vi "Process.vi"(8 "error in (no error)":errorcluster, 10 "Pound in":refnum<class "Pound.lvclass">, 11 "Qbus in":refnum<class "Qbus.lvclass">) -> (0 "error out":errorcluster)   [LabVIEW 2015]
doc: "The Analysis process calculates features and spectral bands, or trends, from waveforms the channels in a data group acquire. After these values are calculated, subsequent processes that evaluate their data to trigger alarms, file collections, and so on can operate."
uses:
  <vilib>/addons/Qbus/Qbus.lvclass
  <vilib>/NI/Software Watchdog/Pound/Pound.lvclass
  <vilib>/addons/InsightCM/Devices/Shared/VibrationAnalysisLoop/controls/Config.ctl
  <vilib>/addons/InsightCM/Devices/Shared/VibrationAnalysisLoop/controls/Group.ctl
  <vilib>/addons/InsightCM/Utilities/Analysis/Shared/controls/Channel.ctl
  <vilib>/addons/InsightCM/Utilities/Analysis/Shared/controls/Feature.ctl
  <vilib>/addons/InsightCM/Utilities/Analysis/Shared/controls/AmplitudeScale.ctl
  <vilib>/addons/InsightCM/Utilities/ChannelStatus/controls/RangeParams.ctl
  <vilib>/addons/InsightCM/Devices/Shared/VibrationAnalysisLoop/VibrationAnalysis.lvlib
  <vilib>/NI/Software Watchdog/Watchdog/Watchdog.lvclass
  <vilib>/addons/InsightCM/Devices/Shared/QbusHelpers/QbusHelper.lvlib
  <vilib>/addons/InsightCM/Devices/Shared/DataFlow/DataFlow.lvlib
  <vilib>/addons/InsightCM/Devices/Shared/TdmsCreator/TdmsCreator.lvlib
  <vilib>/addons/InsightCM/Utilities/Analysis/Shared/AnalysisHelper.lvlib
  <vilib>/addons/InsightCM/Utilities/ChannelStatus/ChannelStatus.lvlib
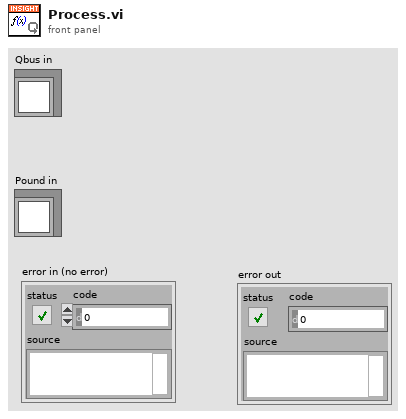
[diagram p1: front panel]
types:
  T1 = typedef "VibrationAnalysis.lvlib/Config.ctl" = cluster{"Groups":T2[]}
  T2 = typedef "VibrationAnalysis.lvlib/Group.ctl" = cluster{"Name":string, "Speed Ref Id":string, "Channels":T3[]}
  T3 = typedef "AnalysisHelper.lvlib/Channel.ctl" = cluster{"Name":string, "Id":string, "Type":string, "Status Tag":string, "Speed Reference":string, "Speed Ratio":dbl, "Pair Channel":string, "Source Channel":string, "Sensitivity":dbl, "Features":T4[], "Data Valid":bool, "Acq Timestamp":timestamp, "RangeCheck":T6}
  T4 = typedef "AnalysisHelper.lvlib/Feature.ctl" = cluster{"MetricType":string, "TdmsPropName":string, "DisplayName":string, "Unit":string, "Use Volts":bool, "Value":dbl, "Tag Id":string, "Properties":variant, "Amplitude Scale":T5}
  T5 = typedef "AnalysisHelper.lvlib/AmplitudeScale.ctl" = enum16{"rms", "peak", "pk-pk"}
  T6 = typedef "ChannelStatus.lvlib/RangeParams.ctl" = cluster{"Enabled":bool, "Max":dbl, "Min":dbl}
  T7 = typedef "TdmsCreator.lvlib/RegisterTrendTdmsPropertiesRoutedMessage.ctl" = cluster{"DataGroup":string, "TdmsGroup":string, "Trends":T8[]}
  T8 = typedef "TdmsCreator.lvlib/Trend.ctl" = cluster{"ChannelName":string, "PointId":string, "TdmsPropName":string, "TdmsDisplayName":string, "TdmsUnitValue":string}
  T9 = typedef "DataFlow.lvlib/Data.ctl" = cluster{"DataGroup":string, "Waveforms":T10, "Map":T11}
  T10 = typedef "wfmSGL_DVR.ctl" = refnum<data-value>
  T11 = typedef "PointValueMap.lvlib/PointMap.ctl" = refnum<data-value>
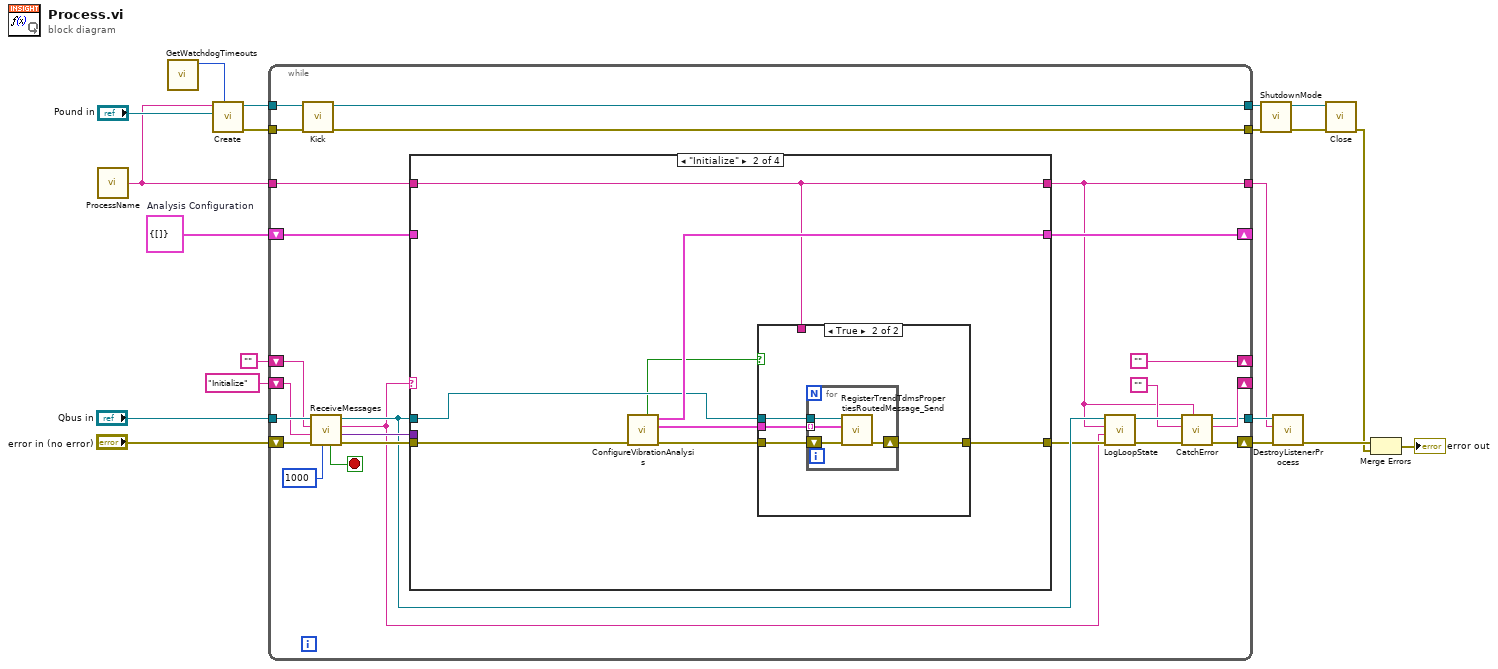
[diagram p0: block diagram]
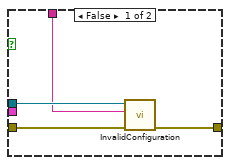
[diagram p3: hidden frame]
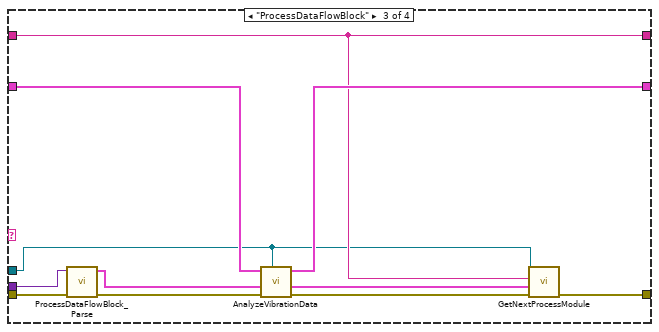
[diagram p4: hidden frame]
diagram:
  w8 = T1 {"Groups"=[]}  # Analysis Configuration
  n1 = call <vilib>:"ProcessName.vi"() -> ("ProcessName"=w13:string)  [unwired: 5 in]
  n2 = call <vilib>:"GetWatchdogTimeouts.vi"() -> ("software timeout"=w1:u32)  [unwired: 10 in, 1 out]
  n3 = call <vilib>:"Create.vi"("Execution Timeout (ms)"=w1, "Pound"="Pound in", "Name"=w13) -> ("error out"=w9:errorcluster, "Watchdog"=w10:refnum<data-value>)  [unwired: 7 in]
  n4 = while {
    shift-right: [""] -> _
    shift-left: "" -> [w40]
    shift-right: [w46] -> _
    shift-left: w8 -> [w45]
    shift-right: [w27] -> _
    shift-left: "Initialize" ("MsgName") -> [w38]
    tunnel: w13 -> [w33]
    tunnel: [w26] -> w16
    tunnel: [w24] -> w15
    tunnel: "Qbus in" -> [w43]
    tunnel: [w37] -> w12
    tunnel: [w36] -> w11
    tunnel: w10 -> [w35]
    tunnel: w9 -> [w34]
    shift-right: [w25] -> w17
    shift-left: "error in (no error)" -> [w39]
    stop <- w22 stop-if-true
    n5 = call <vilib>:"Kick.vi"("error in (no error)"=w34, "Watchdog"=w35) -> ("error out"=w37:errorcluster, "Watchdog"=w36:refnum<data-value>)  [unwired: 8 in]
    n6 = call <vilib>:"ReceiveMessages.vi"("Timeout(100)"=1000, "error in (no error)"=w39, "Priority Action"=w38, "Default Action"=w40, "Qbus in"=w43) -> ("error out"=w41:errorcluster, "MsgValue"=w42:variant, "Action"=w23:string, "Qbus out"=w32:refnum<class "Qbus.lvclass">, "Exit"=w22:bool)  [unwired: 2 in]
    n7 = case shown="\"Initialize\"" w23 {
      tunnel: w41 -> [w49 w53 w78 w82]
      tunnel: [w49 w52 w71 w82] -> w31
      tunnel: w42 -> [_ _ w77 _]
      tunnel: [w48 w57 w79 w81] -> w46
      tunnel: w45 -> [w48 _ w80 w81]
      tunnel: w32 -> [_ w56 w70 _]
      tunnel: [w47 w50 w72 w83] -> w24
      tunnel: w33 -> [w47 w50 w72 w83]
      frame Default {
      }
      frame "Initialize" {
        n8 = call "ConfigureVibrationAnalysis.vi"("error in (no error)"=w53) -> ("error out"=w54:errorcluster, "register trends"=w55:T7[], "analysis config"=w57:T1, "all config found?"=w51:bool)  [unwired: 7 in]
        n9 = case shown="True" w51 {
          tunnel: w56 -> [w61 w65]
          tunnel: w55 -> [_ w64]
          tunnel: w54 -> [w60 w63]
          tunnel: [w59 w62] -> w52
          tunnel: w50 -> [w58 _]
          frame False {
            n10 = call <vilib>:"InvalidConfiguration.vi"("error in (no error)"=w60, "description"=w58, "Qbus in"=w61) -> ("error out"=w59:errorcluster)  [unwired: 7 in, 1 out]
          }
          frame True {
            n11 = for {
              tunnel: w64 -> [w69] mode=indexing
              shift-right: [w67] -> w62
              shift-left: w63 -> [w68]
              tunnel: w65 -> [w66]
              n12 = call <vilib>:"RegisterTrendTdmsPropertiesRoutedMessage_Send.vi"("error in (no error)"=w68, "register trend"=w69, "Qbus in"=w66) -> ("error out"=w67:errorcluster)  [unwired: 7 in, 1 out]
            }
          }
        }
      }
      frame "ProcessDataFlowBlock" {
        n13 = call <vilib>:"ProcessDataFlowBlock_Parse.vi"("error in (no error)"=w78, "body"=w77) -> ("error out"=w74:errorcluster, "data"=w75:T9)  [unwired: 8 in]
        n14 = call <vilib>:"AnalyzeVibrationData.vi"("Qbus in"=w70, "error in (no error)"=w74, "data in"=w75, "Analysis Config"=w80) -> ("error out"=w73:errorcluster, "data out"=w76:T9, "Analysis Config Out"=w79:T1)  [unwired: 5 in]
        n15 = call <vilib>:"GetNextProcessModule.vi"("error in (no error)"=w73, "data"=w76, "source"=w72, "Qbus in"=w70) -> ("error out"=w71:errorcluster)  [unwired: 6 in, 1 out]
      }
      frame "Exit" {
      }
    }
    n16 = call <vilib>:"LogLoopState.vi"("error in (no error)"=w31, "loop action"=w23, "process name"=w24, "Qbus in"=w32) -> ("error out"=w28:errorcluster, "Qbus out"=w30:refnum<class "Qbus.lvclass">)  [unwired: 6 in]
    n17 = call <vilib>:"CatchError.vi"("source"=w24, "error in (no error)"=w28, "next action in"="", "Qbus in"=w30) -> ("error out"=w25:errorcluster, "next action out"=w27:string, "Qbus out"=w26:refnum<class "Qbus.lvclass">)  [unwired: 5 in]
  }
  n18 = call <vilib>:"ShutdownMode.vi"("error in (no error)"=w12, "Watchdog"=w11) -> ("error out"=w18:errorcluster, "Watchdog"=w19:refnum<data-value>)  [unwired: 8 in]
  n19 = call <vilib>:"DestroyListenerProcess.vi"("error in (no error)"=w17, "process name"=w15, "Qbus in"=w16) -> ("error in (no error)"=w7:errorcluster)  [unwired: 7 in, 1 out]
  n20 = call <vilib>:"Close.vi"("error in (no error)"=w18, "Watchdog"=w19) -> ("error out"=w6:errorcluster)  [unwired: 9 in]
  n21 = Merge Errors(w7, w6) -> (→"error out":errorcluster)
